vi "VFH Cost Function.vi"(8 "target heading (relative to current)":dbl, 9 "last commanded heading (relative to current)":dbl, 11 "candidate heading (relative to current)":dbl) -> (3 "cost":dbl)   [LabVIEW 2017, in "NI_Robotics_Vector Field Histogram.lvlib"]
uses:
  <vilib>/robotics/Obstacle Avoidance/Advanced Vector Field Histogram/NI_Robotics_Vector Field Histogram.lvlib
  <vilib>/Analysis/coordinate.llb/Wrap Angle (scalar).vi
  <vilib>/Analysis/NI_AAL_Angle.lvlib
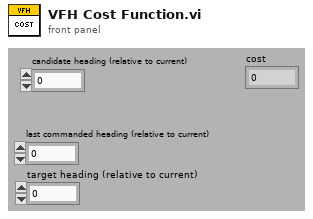
[diagram p1: front panel]
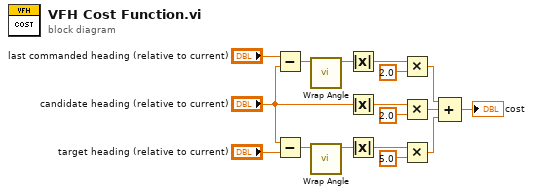
[diagram p0: block diagram]
diagram:
  n1 = Subtract(x="last commanded heading (relative to current)", y="candidate heading (relative to current)") -> (x-y=w4:dbl)
  n2 = Subtract(x="candidate heading (relative to current)", y="target heading (relative to current)") -> (x-y=w2:dbl)
  n3 = call-poly <vilib>:"Wrap Angle.vi"("angle in"=w4) -> ("angle out"=w3:dbl)  [unwired: 9 in, 1 out]
  n4 = call-poly <vilib>:"Wrap Angle.vi"("angle in"=w2) -> ("angle out"=w1:dbl)  [unwired: 9 in, 1 out]
  n5 = Absolute Value(x=w3) -> (abs(x)=w15:dbl)
  n6 = Absolute Value(x="candidate heading (relative to current)") -> (abs(x)=w10:dbl)
  n7 = Absolute Value(x=w1) -> (abs(x)=w6:dbl)
  n8 = Multiply(x=w15, y=2.0 ("x")) -> (x*y=w17:dbl)
  n9 = Multiply(x=w10, y=2.0) -> (x*y=w11:dbl)
  n10 = Multiply(x=w6, y=5.0) -> (x*y=w8:dbl)
  n11 = Compound Arithmetic op=ADD(w17, w11, w8) -> (→"cost":dbl)
